vi "GUI_Magspec_BELLA.vi"() -> ()   [LabVIEW 2013]
uses:
  shared programs/GUI_Template/GUI_master/tcp_new_data_event.ctl
  shared programs/GUI_Template/GUI_master/tcp new data cluster.ctl
  shared programs/MySQL/Preset Query Enum.ctl
  <vilib>/Analysis/2dsp.llb/Decimate (single shot, DBL).vi
  <vilib>/Utility/tcp.llb/UDP Multicast Read-Only Open.vi
  <vilib>/vision/NI_Vision_Development_Module.lvlib
  <vilib>/Analysis/NI_AALPro.lvlib
panel:
  out "ShotNumber":i32
  out "data":string[][](array[string])
  in  "rank for LPF":i32=2
  out "Waveform Graph":dbl[](graph)
  in  "HorizontalLineout::12":dbl[](array[numeric]) caption="HorizontalLineout MagSpecA"
  in  "HorizontalLineout::11":dbl[](array[numeric]) caption="HorizontalLineout MagSpecA"
  in  "HorizontalLineout::10":dbl[](array[numeric]) caption="HorizontalLineout MagSpecA"
  in  "HorizontalLineout::9":dbl[](array[numeric]) caption="HorizontalLineout MagSpecA"
  in  "HorizontalLineout::8":dbl[](array[numeric]) caption="HorizontalLineout MagSpecA"
  in  "HorizontalLineout::7":dbl[](array[numeric]) caption="HorizontalLineout MagSpecA"
  in  "HorizontalLineout::6":dbl[](array[numeric]) caption="HorizontalLineout MagSpecA"
  in  "HorizontalLineout::5":dbl[](array[numeric]) caption="HorizontalLineout MagSpecA"
  in  "HorizontalLineout::4":dbl[](array[numeric]) caption="HorizontalLineout MagSpecA"
  in  "HorizontalLineout::3":dbl[](array[numeric]) caption="HorizontalLineout MagSpecA"
  in  "HorizontalLineout::2":dbl[](array[numeric]) caption="HorizontalLineout MagSpecA"
  in  "HorizontalLineout::1":dbl[](array[numeric]) caption="HorizontalLineout MagSpecA"
  in  "GUIdevice 12":string="MagSpecL"
  in  "GUIdevice 11":string="MagSpecK"
  in  "GUIdevice 10":string="MagSpecJ"
  in  "GUIdevice 9":string="MagSpecI"
  in  "GUIdevice 8":string="MagSpecH"
  in  "GUIdevice 7":string="MagSpecG"
  in  "GUIdevice 6":string="MagSpecF"
  in  "GUIdevice 5":string="MagSpecE"
  in  "GUIdevice 4":string="MagSpecD"
  in  "GUIdevice 3":string="MagSpecC"
  in  "GUIdevice 2":string="MagSpecB"
  in  "GUIdevice 1":string="MagSpecA"
  in  "GUIdevice 14":string="BELLA_HallProbe"
  out "error IO 2":errorcluster
  out "tcp data event":T1
  out "Momentum 14":dbl=0.0055371 caption="Momentum (GeV/c)" min=0.0 max=0.0 format="%#.1f"
  out "Momentum 13":dbl=0.06921375 caption="Momentum (GeV/c)" min=0.0 max=0.0 format="%#.1f"
  out "Momentum 12":dbl=0.276855 caption="Momentum (GeV/c)" min=0.0 max=0.0 format="%#.1f"
  out "Momentum 11":dbl=0.67829475 caption="Momentum (GeV/c)" min=0.0 max=0.0 format="%#.1f"
  out "Momentum 10":dbl=1.218162 caption="Momentum (GeV/c)" min=0.0 max=0.0 format="%#.1f"
  out "Momentum 9":dbl=2.0210415 caption="Momentum (GeV/c)" min=0.0 max=0.0 format="%#.1f"
  out "Momentum 8":dbl=2.97619125 caption="Momentum (GeV/c)" min=0.0 max=0.0 format="%#.1f"
  out "Momentum 7":dbl=4.014397499999999 caption="Momentum (GeV/c)" min=0.0 max=0.0 format="%#.1f"
  out "Momentum 6":dbl=4.36046625 caption="Momentum (GeV/c)" min=0.0 max=0.0 format="%#.1f"
  out "Momentum 5":dbl=5.675527499999999 caption="Momentum (GeV/c)" min=0.0 max=0.0 format="%#.1f"
  out "Momentum 4":dbl=7.19823 caption="Momentum (GeV/c)" min=0.0 max=0.0 format="%#.1f"
  out "Momentum 3":dbl=8.582505 caption="Momentum (GeV/c)" min=0.0 max=0.0 format="%#.1f"
  out "Momentum 2":dbl=9.5514975 caption="Momentum (GeV/c)" min=0.0 max=0.0 format="%#.1f"
  out "Momentum 1":dbl=26.301225 caption="Momentum (GeV/c)" min=0.0 max=0.0 format="%#.1f"
  in  "Field::14":dbl=2.76855 caption="Magnetic Field (mT)" min=0.0 max=0.0 format="%_4f"
  out "Boolean":bool
  out "EBeam":T2(plugin-control) caption="Beam Profile"
  out "L":T2(plugin-control) caption="L Cam"
  out "K":T2(plugin-control) caption="K Cam"
  out "J":T2(plugin-control) caption="J Cam"
  out "I":T2(plugin-control) caption="I Cam"
  out "H":T2(plugin-control) caption="H Cam"
  out "G":T2(plugin-control) caption="G Cam"
  out "F":T2(plugin-control) caption="F Cam"
  out "E":T2(plugin-control) caption="E Cam"
  out "B":T2(plugin-control) caption="B Cam"
  out "A":T2(plugin-control) caption="A Cam"
  out "D":T2(plugin-control) caption="D Cam"
  out "C":T2(plugin-control) caption="C cam"
  in  "stop":bool
  # "AA side"
  # "T\no\np"
  # "B\nT\nM"
  # "Parking side"
  # "Beam Axis"
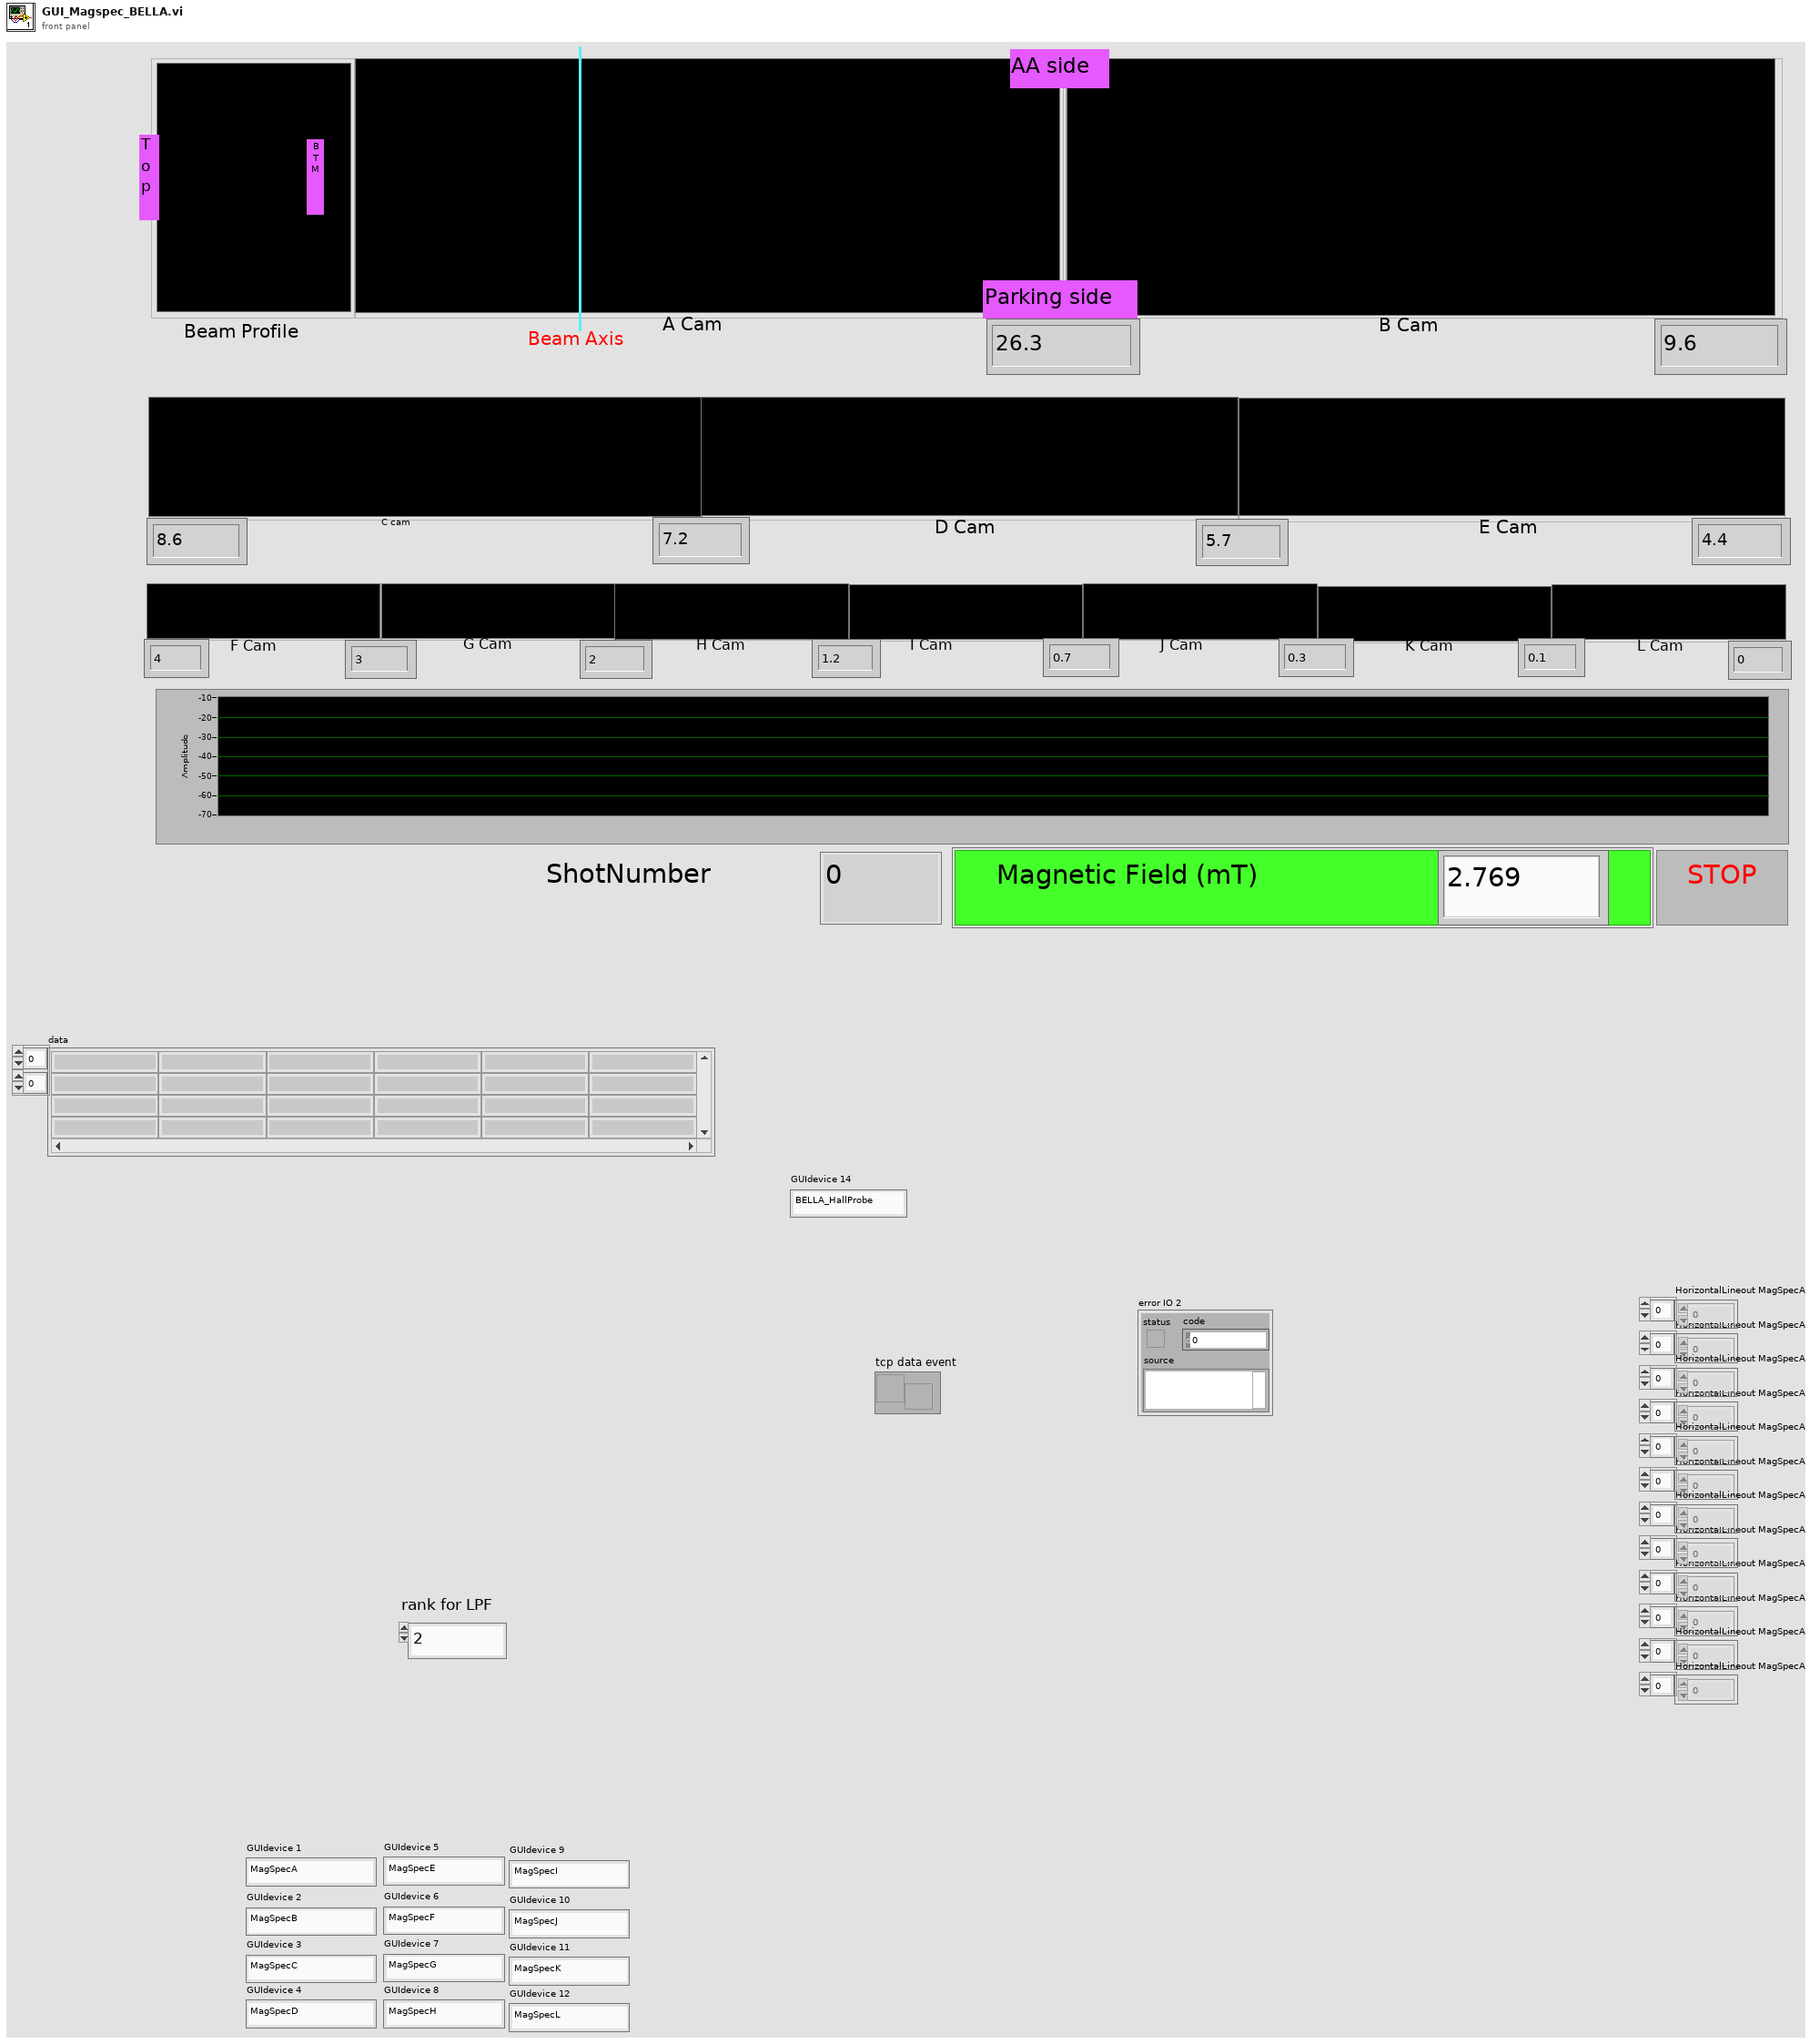
[diagram p1: front panel]
types:
  T1 = typedef "tcp_new_data_event.ctl" = refnum<user-event>
  T2 = typedef "IMAQ Image.ctl" = refnum<image>
  T3 = typedef "Image Type" = u32
  T4 = typedef "Preset Query Enum.ctl" = enum16{"Get Locations", "Get all IPs and MACs", "Get classes", "Get expt variables to set at scanstart for particular device", "Get expt devices and variables with start values", "Get expt devices and variables (with data to get)", "Get expt devices with data to get", "Get Expt devices and GUIs", "Get all devices basic properties", "Get Virtual Devices Core Info", "Get Expt names", "Get experiment basic properties", "Get experiment alarm variables", "Get MC Ports", "Get device network comm port", "Get devicetype lvclass path", "Get basic device properties", "Get Init Order", "Get all setable variables of a device", "Get device variable aliases", "Get force values of all settable variables", "Get all variables of a devicetype", "Get all variables of a device", "Get plotter details", "Get Saved Scans", "Get Scan Info", "GetGeneralGUIs", "Get expt for plotter", "Get plotter IDs from expt", "Get all devices", "Get all Virtual Devices", "Get variable and device info for Virtual Device", "GetItemLocatorIP", "Get IPs for GUIs", "Get DeviceType from Device", "GetLocalPortRange", "GetDevicePresetVariables", "Get Device Configuration", "GetAllPresetNames", "GetAllConfigurationNames", "GetPresetDeviceNames"}
  T5 = typedef "tcp new data cluster.ctl" = cluster{"EventEnum":enum16{"new data", "connection status update"}, "Device name":string}
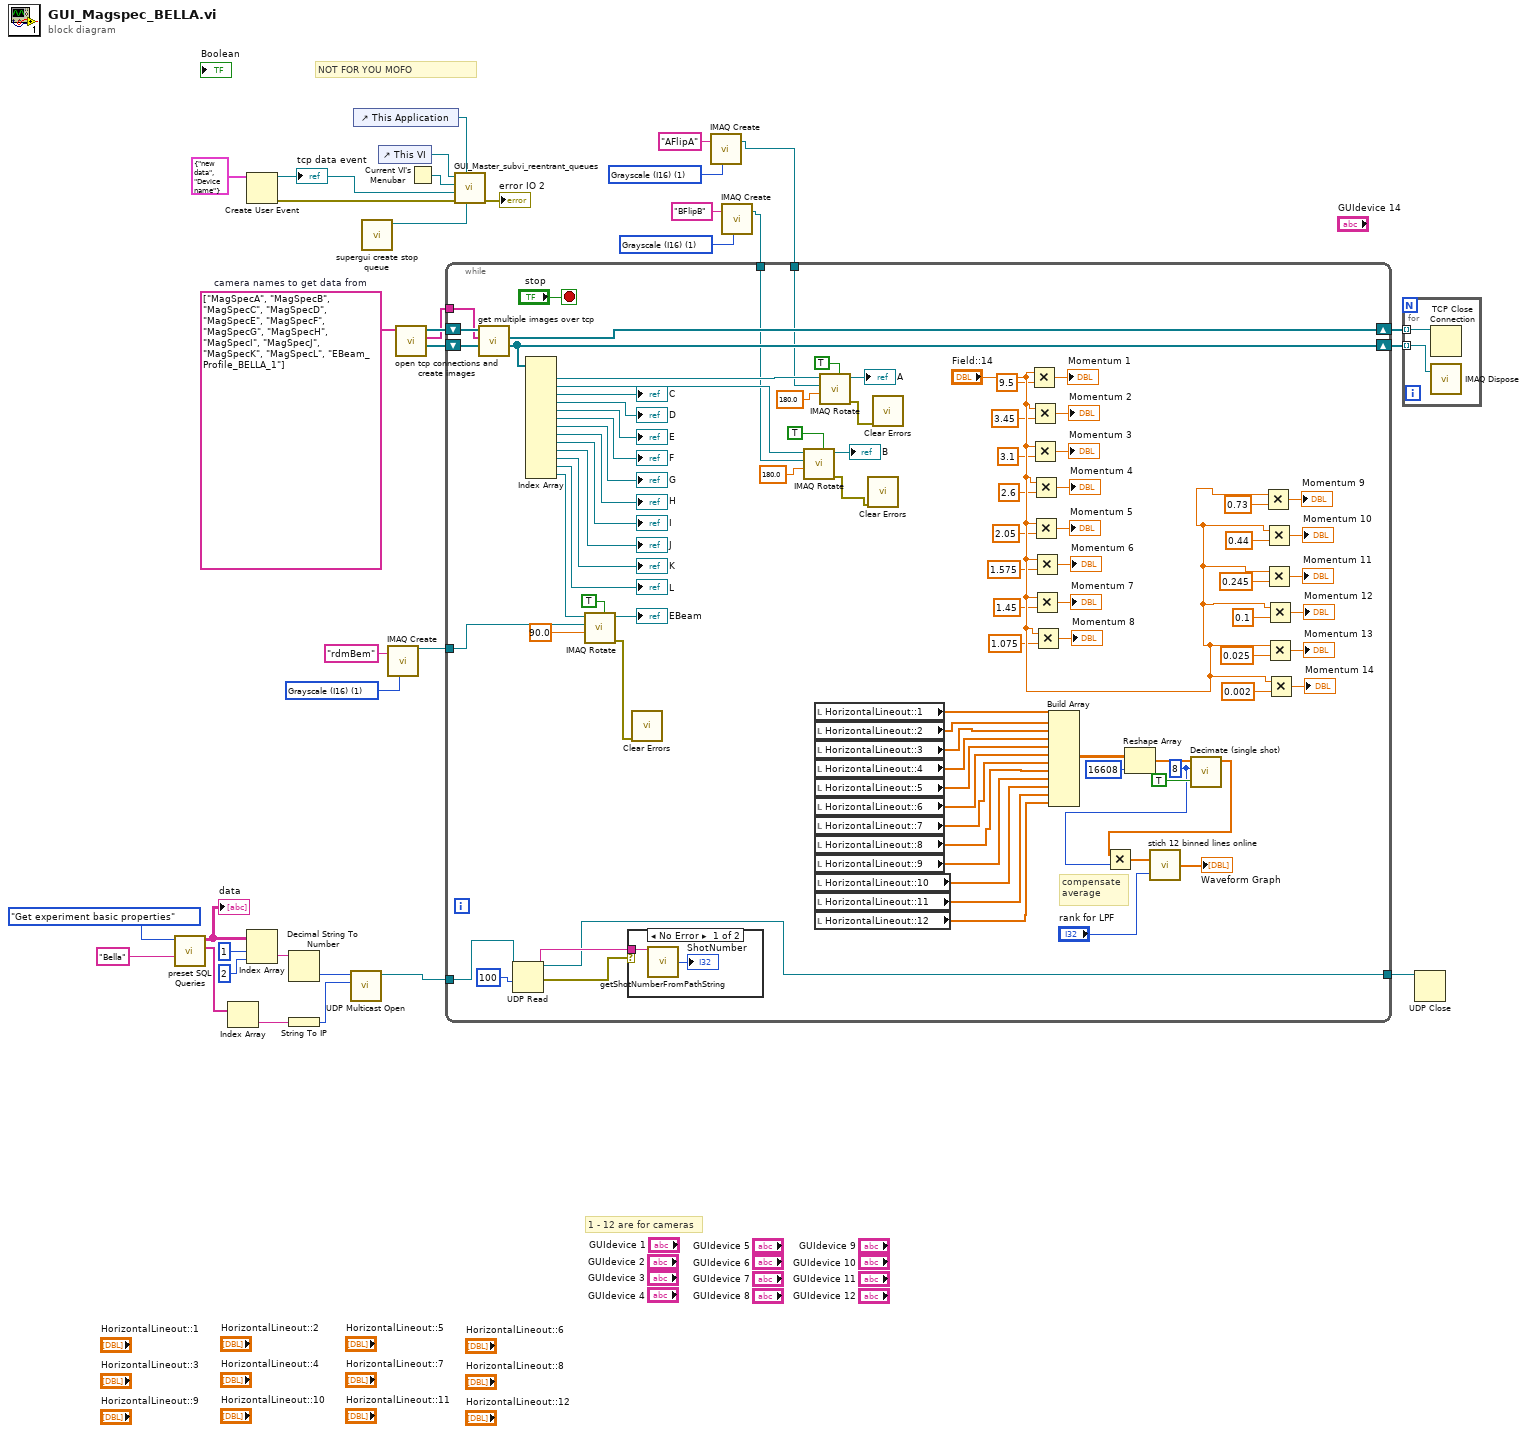
[diagram p0: block diagram]
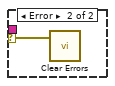
[diagram p2: hidden frame]
diagram:
  w3 = T3 1 items=["Grayscale (U8)", "Grayscale (I16)", "Grayscale (SGL)", "Complex (CSG)", "RGB (U32)", "HSL (U32)", "RGB (U64)", "Grayscale (U16)"] ("Image Type")
  w7 = T3 1 items=["Grayscale (U8)", "Grayscale (I16)", "Grayscale (SGL)", "Complex (CSG)", "RGB (U32)", "HSL (U32)", "RGB (U64)", "Grayscale (U16)"] ("Image Type")
  w9 = T3 1 items=["Grayscale (U8)", "Grayscale (I16)", "Grayscale (SGL)", "Complex (CSG)", "RGB (U32)", "HSL (U32)", "RGB (U64)", "Grayscale (U16)"] ("Image Type")
  w32 = string[] ["MagSpecA", "MagSpecB", "MagSpecC", "MagSpecD", "MagSpecE", "MagSpecF", "MagSpecG", "MagSpecH", "MagSpecI", "MagSpecJ", "MagSpecK", "MagSpecL", "EBeam_Profile_BELLA_1"]  # camera names to get data from
  # "1 - 12 are for cameras"
  # "NOT FOR YOU MOFO"
  n1 = call "preset SQL Queries.vi"("Expt name / MCIP/ Variable/Preset Name"="Bella", "Preset Query"=Preset_Query_Enum."Get experiment basic properties") -> ("1st column 1st data"=w15:string[], "data"=w16:string[][])  [unwired: 7 in, 1 out]
  "data" <- w16
  n2 = Index Array(array=w15) -> (element=w14:string)  [unwired: 1 in]
  n3 = Create User Event(user event datatype=T5 {"EventEnum"=enum."new data", "Device name"="Device name"} ("New Event")) -> (user event=w24:refnum<user-event>, error out=w25:errorcluster)  [unwired: 1 in]
  "tcp data event" <- w24
  n4 = Index Array(array=w16, index (row)=1, index (col)=2 ("disabled index (col)")) -> (element=w17:string)
  n5 = Decimal String To Number(string=w17) -> (number=w13:i32)  [unwired: 2 in, 1 out]
  n6 = String To IP(1:w14) -> (0:w20:u32)
  n7 = call-poly <vilib>:"UDP Multicast Open.vi"("multicast addr"=w20, "port"=w13) -> ("connection ID"=w12:refnum<k16>)  [unwired: 7 in, 2 out]
  n8 = control-ref of="This Application"() -> (w23:refnum<vi>)
  n9 = call "supergui create stop queue.vi"() -> ("STOP Queue out"=w1:refnum<queue>)  [unwired: 11 in]
  n10 = control-ref of="This VI"() -> (w28:refnum<vi>)
  n11 = call "IMAQ Create"("Image Name"="rdmBem", "Image Type"=w3) -> ("New Image"=w2:T2)  [unwired: 3 in, 1 out]
  n12 = call "open tcp connections and create images.vi"("devices to get data from"=w32) -> ("images"=w31:T2[], "subscribe messages\nfor process vis"=w33:string[], "tcp connections"=w34:refnum<k5>[])  [unwired: 8 in]
  n13 = Current VI's Menubar() -> (w27:refnum<k9>)
  n14 = call "GUI_Master_subvi_reentrant_queues.vi"("STOP Queue in"=w1, "This Application"=w23, "error in (no error)"=w25, "tcp data event"=w24, "Caller menu reference"=w27, "Caller VI ref"=w28) -> ("error out"=→"error IO 2":errorcluster)  [unwired: 5 in]
  n15 = call "IMAQ Create"("Image Name"="AFlipA", "Image Type"=w9) -> ("New Image"=w8:T2)  [unwired: 3 in, 1 out]
  n16 = call "IMAQ Create"("Image Name"="BFlipB", "Image Type"=w7) -> ("New Image"=w5:T2)  [unwired: 3 in, 1 out]
  n17 = while {
    shift-right: [w122] -> w35
    shift-left: w34 -> [w123]
    tunnel: w33 -> [w121]
    shift-right: [w119] -> w30
    shift-left: w31 -> [w120]
    tunnel: w12 -> [w40]
    tunnel: [w39] -> w11
    tunnel: w8 -> [w38]
    tunnel: w5 -> [w37]
    tunnel: w2 -> [w36]
    stop <- "stop" stop-if-true
    w45 = 8 ("decimating factor")
    # "compensate\naverage"
    n18 = call "get multiple images over tcp.vi"("images In"=w120, "subscribeMessages"=w121, "TCP_Refs In"=w123) -> ("Images out"=w119:T2[], "TCP_Refs_out"=w122:refnum<k5>[])  [unwired: 4 in, 3 out]
    n19 = UDP Read(connection ID=w40, timeout ms (25000)=100) -> (data out=w42:string, error out=w41:errorcluster, 3:w39:refnum<k16>)  [unwired: 1 in, 3 out]
    n20 = Index Array(array=w119) -> (element #1=w98:T2, element #2=w103:T2, element #3=→"C":T2, element #4=→"D":T2, element #5=→"E":T2, element #6=→"F":T2, element #7=→"G":T2, element #8=→"H":T2, element #9=→"I":T2, element #10=→"J":T2, element #11=→"K":T2, element #12=→"L":T2, element #13=w107:T2)  [unwired: 13 in]
    n21 = call "IMAQ Rotate"("Maintain Size"=TRUE, "Angle (degrees)"=sgl 90.0, "Image Dst"=w36, "Image Src"=w107) -> ("error out"=w96:errorcluster, "Image Dst Out"=→"EBeam":T2)  [unwired: 6 in]
    n22 = case shown="No Error" w41 {
      selector: w41 -> [_ w127]
      tunnel: w42 -> [w126 _]
      frame No Error {
        n23 = call "getShotNumberFromPathString.vi"("Path String"=w126) -> ("ShotNumber from path"=→"ShotNumber":i32)
      }
      frame Error {
        n24 = call <vilib>:"Clear Errors.vi"("error in (no error)"=w127) -> ()  [unwired: 6 in, 1 out]
      }
    }
    n25 = call <vilib>:"Clear Errors.vi"("error in (no error)"=w96) -> ()  [unwired: 6 in, 1 out]
    n26 = call "IMAQ Rotate"("Maintain Size"=TRUE, "Angle (degrees)"=sgl 180.0, "Image Dst"=w37, "Image Src"=w103) -> ("error out"=w95:errorcluster, "Image Dst Out"=→"B":T2)  [unwired: 6 in]
    n27 = local read "HorizontalLineout::1"() -> (w64:dbl[])
    n28 = local read "HorizontalLineout::2"() -> (w63:dbl[])
    n29 = local read "HorizontalLineout::3"() -> (w62:dbl[])
    n30 = local read "HorizontalLineout::4"() -> (w61:dbl[])
    n31 = local read "HorizontalLineout::5"() -> (w60:dbl[])
    n32 = local read "HorizontalLineout::6"() -> (w59:dbl[])
    n33 = local read "HorizontalLineout::7"() -> (w58:dbl[])
    n34 = local read "HorizontalLineout::8"() -> (w57:dbl[])
    n35 = local read "HorizontalLineout::9"() -> (w56:dbl[])
    n36 = local read "HorizontalLineout::10"() -> (w55:dbl[])
    n37 = local read "HorizontalLineout::11"() -> (w54:dbl[])
    n38 = local read "HorizontalLineout::12"() -> (w53:dbl[])
    n39 = call "IMAQ Rotate"("Maintain Size"=TRUE, "Angle (degrees)"=sgl 180.0, "Image Dst"=w38, "Image Src"=w98) -> ("error out"=w94:errorcluster, "Image Dst Out"=→"A":T2)  [unwired: 6 in]
    n40 = call <vilib>:"Clear Errors.vi"("error in (no error)"=w95) -> ()  [unwired: 6 in, 1 out]
    n41 = call <vilib>:"Clear Errors.vi"("error in (no error)"=w94) -> ()  [unwired: 6 in, 1 out]
    n42 = Multiply(x="Field::14", y=9.5) -> (x*y=→"Momentum 1":dbl)
    n43 = Multiply(x="Field::14", y=3.45) -> (x*y=→"Momentum 2":dbl)
    n44 = Multiply(x="Field::14", y=3.1) -> (x*y=→"Momentum 3":dbl)
    n45 = Multiply(x="Field::14", y=2.6) -> (x*y=→"Momentum 4":dbl)
    n46 = Multiply(x="Field::14", y=2.05) -> (x*y=→"Momentum 5":dbl)
    n47 = Multiply(x="Field::14", y=1.575) -> (x*y=→"Momentum 6":dbl)
    n48 = Multiply(x="Field::14", y=1.45) -> (x*y=→"Momentum 7":dbl)
    n49 = Multiply(x="Field::14", y=1.075) -> (x*y=→"Momentum 8":dbl)
    n50 = Build Array(w64, w63, w62, w61, w60, w59, w58, w57, w56, w55, w54, w53) -> (w52:dbl[][])
    n51 = Reshape Array(w52, 16608 ("dimension size")) -> (w50:dbl[])
    n52 = call-poly <vilib>:"Decimate (single shot).vi"("averaging"=TRUE, "decimating factor"=w45, "X"=w50) -> ("Decimated Array"=w46:dbl[])  [unwired: 7 in, 1 out]
    n53 = Multiply(x=w46, y=w45) -> (x*y=w47:dbl[])
    n54 = call "stich 12 binned lines online.vi"("rank"="rank for LPF", "Input"=w47) -> ("stiched signal"=→"Waveform Graph":dbl[])
    n55 = Multiply(x="Field::14", y=0.73) -> (x*y=→"Momentum 9":dbl)
    n56 = Multiply(x="Field::14", y=0.44) -> (x*y=→"Momentum 10":dbl)
    n57 = Multiply(x="Field::14", y=0.245) -> (x*y=→"Momentum 11":dbl)
    n58 = Multiply(x="Field::14", y=0.1) -> (x*y=→"Momentum 12":dbl)
    n59 = Multiply(x="Field::14", y=0.025) -> (x*y=→"Momentum 13":dbl)
    n60 = Multiply(x="Field::14", y=0.002) -> (x*y=→"Momentum 14":dbl)
  }
  n61 = for {
    tunnel: w35 -> [w129] mode=indexing
    tunnel: w30 -> [w128] mode=indexing
    n62 = TCP Close Connection(connection ID=w129) -> ()  [unwired: 2 in, 2 out]
    n63 = call "IMAQ Dispose"("Image"=w128) -> ()  [unwired: 5 in, 1 out]
  }
  n64 = UDP Close(connection ID=w11) -> ()  [unwired: 1 in, 2 out]
